vi "Do.vi"(6 "Input":variant, 8 "error in":errorcluster, 9 "Self Enqueuer":refnum<class "Message Enqueuer.lvclass">, 10 "Series Enqueuer":refnum<class "Message Enqueuer.lvclass">, 11 "Task Base in":refnum<class "Task Base.lvclass">) -> (0 "error out":errorcluster, 3 "Task Base out":refnum<class "Task Base.lvclass">)   [LabVIEW 2023, in "HAL GOOP4.lvlib" / "Task Base.lvclass"]
uses:
  Task Base.lvclass
  <vilib>/ActorFramework/Message Enqueuer/Message Enqueuer.lvclass
  <vilib>/Utility/error.llb/Error Cluster From Error Code.vi
  <vilib>/ErrorRing/Error Ring.xnode
  Task Base.lvclass/Task Base.ctl
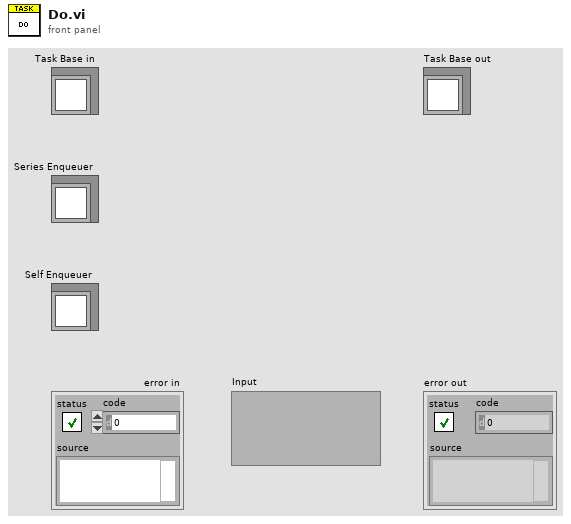
[diagram p1: front panel]
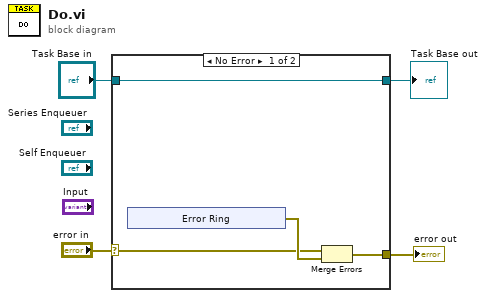
[diagram p0: block diagram]
diagram:
  n1 = case shown="No Error" "error in" {
    selector: "error in" -> [w5 w15]
    tunnel: [w8 w15] -> w4
    tunnel: "Task Base in" -> [w6 w14]
    tunnel: [w6 w14] -> w2
    frame No Error {
      n2 = xnode "Error Ring"() -> ("error out"=w7:errorcluster)
      n3 = Merge Errors(w5, w7) -> (w8:errorcluster)
    }
    frame Error {
    }
  }
  "error out" <- w4
  "Task Base out" <- w2
